vi "SbigRescale.vi"(1 "Window":T1, 2 "Binning Mode":u16, 3 "Image In":i32[][](array[numeric]), 8 "error out 2":errorcluster caption="error in") -> (0 "Image Out":i32[][](array[numeric]), 5 "error out":errorcluster)   [LabVIEW 2009]
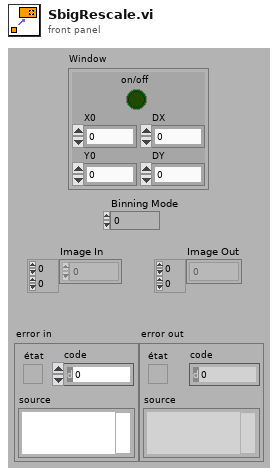
[diagram p1: front panel]
types:
  T1 = cluster{"X0":u16, "Y0":u16, "DX":u16, "DY":u16, "on/off":bool}
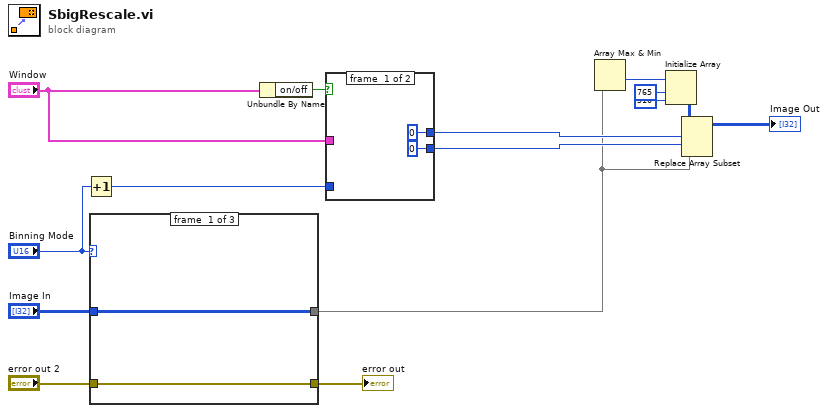
[diagram p0: block diagram]
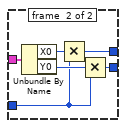
[diagram p2: hidden frame]
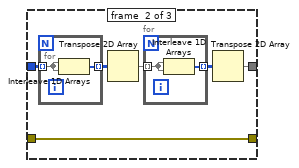
[diagram p3: hidden frame]
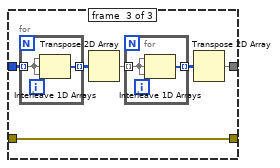
[diagram p4: hidden frame]
diagram:
  n1 = Increment(x="Binning Mode") -> (x+1=w2:u16)
  n2 = case shown="2" "Binning Mode" {
    tunnel: "Image In" -> [w17 w23 w33]
    tunnel: [w17 w19 w29] -> w3
    tunnel: "error out 2" -> [w16 w18 w28]
    tunnel: [w16 w18 w28] -> w15
    frame #0 {
    }
    frame #1 {
      n3 = for {
        tunnel: w23 -> [w26] mode=indexing
        tunnel: [w27] -> w22 mode=indexing
        n4 = Interleave 1D Arrays(w26, w26) -> (w27:i32[])
      }
      n5 = Transpose 2D Array(2D array=w22) -> (transposed array=w21:i32[][])
      n6 = for {
        tunnel: w21 -> [w24] mode=indexing
        tunnel: [w25] -> w20 mode=indexing
        n7 = Interleave 1D Arrays(w24, w24) -> (w25:i32[])
      }
      n8 = Transpose 2D Array(2D array=w20) -> (transposed array=w19:i32[][])
    }
    frame #2 {
      n9 = for {
        tunnel: w33 -> [w36] mode=indexing
        tunnel: [w37] -> w32 mode=indexing
        n10 = Interleave 1D Arrays(w36, w36, w36) -> (w37:i32[])
      }
      n11 = Transpose 2D Array(2D array=w32) -> (transposed array=w31:i32[][])
      n12 = for {
        tunnel: w31 -> [w34] mode=indexing
        tunnel: [w35] -> w30 mode=indexing
        n13 = Interleave 1D Arrays(w34, w34, w34) -> (w35:i32[])
      }
      n14 = Transpose 2D Array(2D array=w30) -> (transposed array=w29:i32[][])
    }
  }
  "error out" <- w15
  n15 = Unbundle By Name("Window") -> ("on/off"=w7:bool)
  n16 = case shown="False" w7 {
    tunnel: [u16 0 w43] -> w10
    tunnel: [u16 0 w42] -> w9
    tunnel: "Window" -> [_ w41]
    tunnel: w2 -> [_ w40]
    frame #0 {
    }
    frame #1 {
      n17 = Unbundle By Name(w41) -> ("X0"=w45:u16, "Y0"=w44:u16)
      n18 = Multiply(x=w45, y=w40) -> (x*y=w43:u16)
      n19 = Multiply(x=w44, y=w40) -> (x*y=w42:u16)
    }
  }
  n20 = Array Max & Min(array=w3) -> (min value=w6:i32)  [unwired: 3 out]
  n21 = Initialize Array(w6, 765 ("Taille de la dimension"), 510 ("Taille de la dimension")) -> (w8:i32[][])
  n22 = Replace Array Subset(array=w8, new element=w3, index (row)=w10, index (col)=w9) -> (→"Image Out":i32[][])
